vi "scale active channels.vi"(9 "input cluster":T1={"Parameters"={"FPGA Ref"=refnum, "data stream"={"data writer name"="error writer", "NS write buffer size"=16, "NS Buffer length"=0}, "FIFO Depth"=0, "Channel controls"={"FIFO channel count"=0, "active indices"=[], "active channels"=0, "channelScaling"=[], "scanivalveCount"=0, "channels"=[]}, "safetyChannels"={"oilP"=0, "airP"=0, "water"=0, "channelLimits"=[]}, "speedChannel"=0, "maxSpeedLimit"=0.0, "Torque"={"fixedOffset"=0.0, "filter"=FALSE, "fallingEdge"=FALSE, "swapEncoders"=FALSE}}, "Variables"={"Intermediary buffer"=[], "buffer position"=0, "write loop counter"=0, "NS write trigger"=0, "NS Connection status"=FALSE, "waiting for NS"=FALSE, "labAmbient"={"pressure"=0.0, "temperature"=0.0}, "scanivalvePorts"=[], "scanivalvePressures"=[], "data stream"="", "activeChannelLimitIndex"=[], "runningSpeedLimit"=0.0, "speedChannelIndex"=0, "Interlocks"={"gearboxOil"=FALSE, "bearingOil"=FALSE, "gearboxAir"=FALSE}, "interlockChannels"={"gearboxOil"=0, "bearingOil"=0, "air"=0}, "limitStates"=[]}}, 11 "raw data":sgl[](array[numeric])) -> (1 "data length":i32, 3 "Active channels":dbl[][](array[numeric]))   [LabVIEW 2018]
uses:
  Type Defs/Data processing loop data.ctl
  Type Defs/FPGA reference.ctl
  PC/type defs/channelControl.ctl
  Type Defs/channelScalingTypes.ctl
  Type Defs/scalingMethods.ctl
  ICL-LabVIEW_General/data channels/parent class/Data Channel.lvclass
  PC/type defs/channelLimitControl.ctl
  PC/type defs/limitActions.ctl
  ICL-LabVIEW_General/data channels/parent class/dataSource.ctl
  ICL-LabVIEW_General/data channels/data channels.lvlib
panel:
  out "time":dbl
  out "Data received":sgl[][](array[numeric])
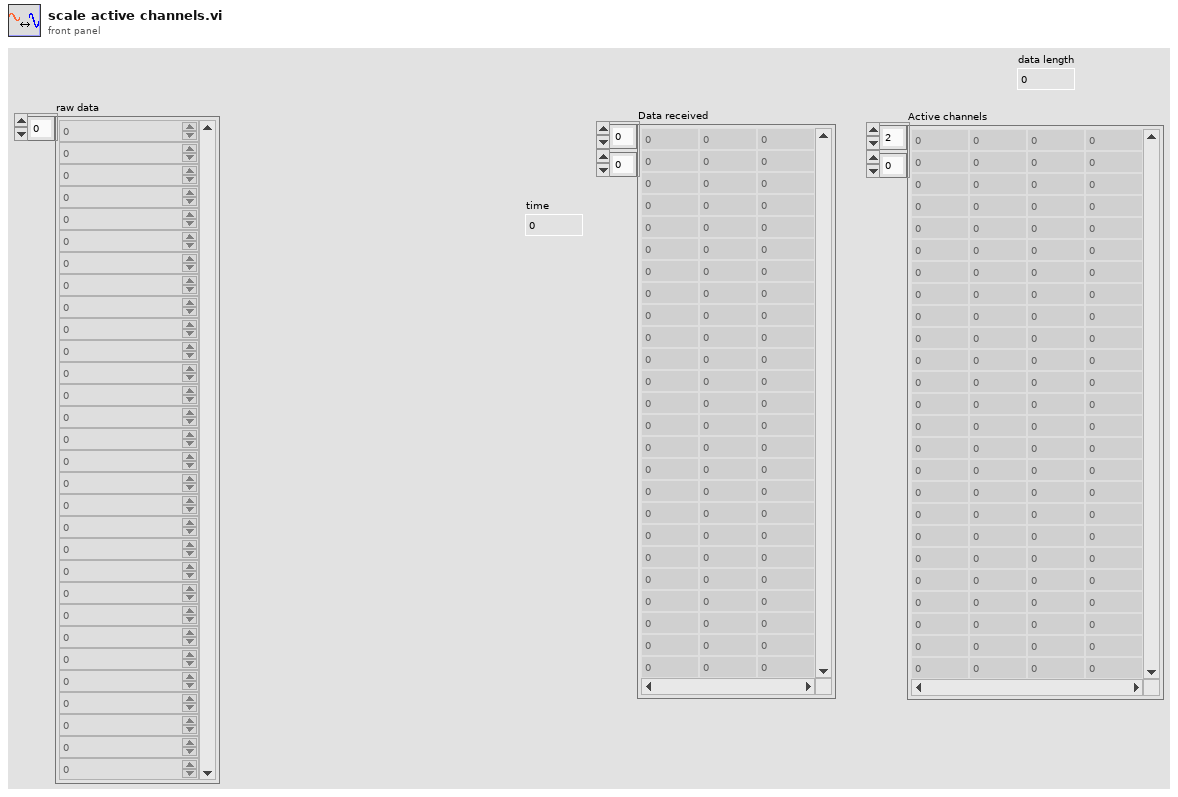
[diagram p1: front panel]
types:
  T1 = typedef "Data processing loop data.ctl" = cluster{"Parameters":cluster{"FPGA Ref":T2, "data stream":cluster{"data writer name":string, "NS write buffer size":i32, "NS Buffer length":u32}, "FIFO Depth":u32, "Channel controls":cluster{"FIFO channel count":i32, "active indices":i16[], "active channels":i32, "channelScaling":T3[], "scanivalveCount":i32, "channels":refnum<class "Data Channel.lvclass">[]}, "safetyChannels":cluster{"oilP":u16, "airP":u16, "water":u16, "channelLimits":T6[]}, "speedChannel":i32, "maxSpeedLimit":dbl, "Torque":cluster{"fixedOffset":dbl, "filter":bool, "fallingEdge":bool, "swapEncoders":bool}}, "Variables":cluster{"Intermediary buffer":dbl[][], "buffer position":u32, "write loop counter":u16, "NS write trigger":u32, "NS Connection status":bool, "waiting for NS":bool, "labAmbient":cluster{"pressure":dbl, "temperature":dbl}, "scanivalvePorts":u16[], "scanivalvePressures":dbl[], "data stream":refnum<k21>, "activeChannelLimitIndex":u16[], "runningSpeedLimit":dbl, "speedChannelIndex":i32, "Interlocks":cluster{"gearboxOil":bool, "bearingOil":bool, "gearboxAir":bool}, "interlockChannels":cluster{"gearboxOil":i32, "bearingOil":i32, "air":i32}, "limitStates":cluster{"warn":bool, "alarm":bool}[]}}
  T2 = typedef "FPGA reference.ctl" = refnum<k20>
  T3 = typedef "channelControl.ctl" = cluster{"index":u16, "active":bool, "channelType":T4, "module":u16, "terminal":u16, "channelName":string, "scalingMethod":T5, "scalingParameters":dbl[], "scaledUnits":string, "tempOffset":dbl}
  T4 = typedef "channelScalingTypes.ctl" = enum16{"calculation", "measurement", "scanivalve", "output", "digital"}
  T5 = typedef "scalingMethods.ctl" = enum16{"none", "linear", "thermocouple", "polynomial", "encoder", "RTD"}
  T6 = typedef "channelLimitControl.ctl" = cluster{"channelID":u16, "Enabled":bool, "warnValue":dbl, "limitValue":dbl, "Invert":bool, "limitAction":T7}
  T7 = typedef "limitActions.ctl" = enum16{"stop", "shutdown", "ignore"}
  T8 = typedef "data channels.lvlib/Data Channel.lvclass/dataSource.ctl" = enum16{"Not available", "FIFO", "Scanivalve", "Remote", "Calculated"}
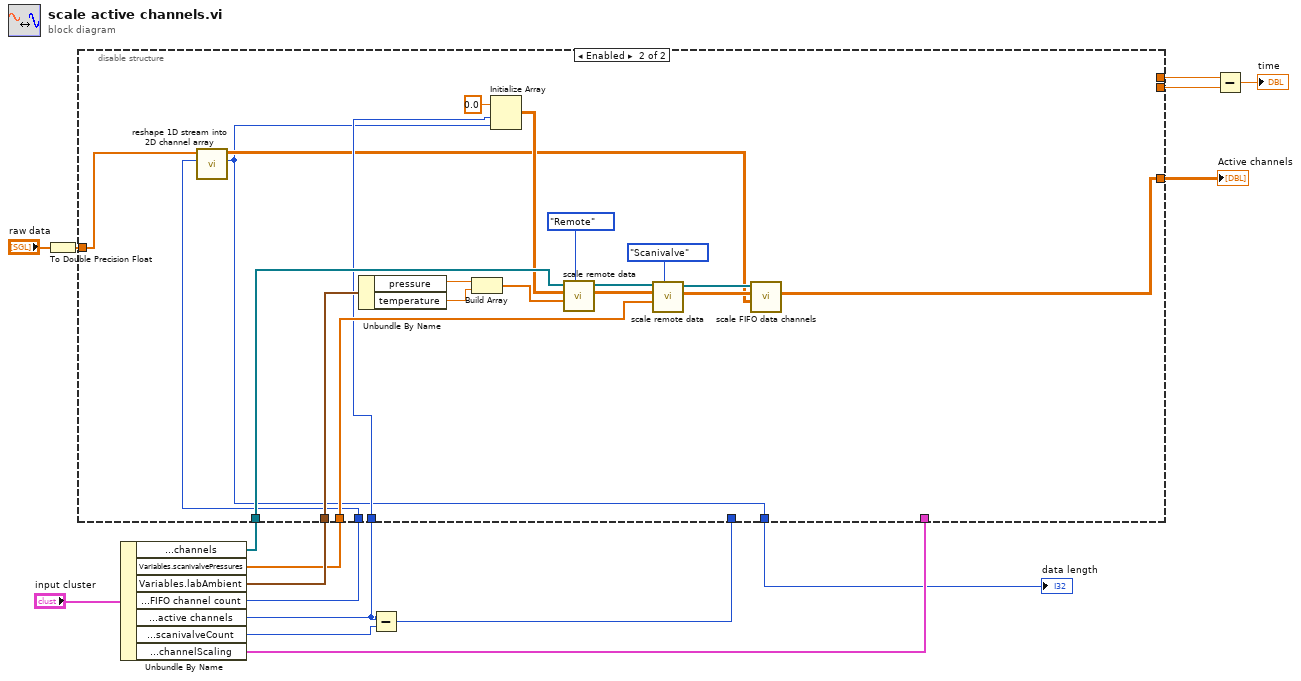
[diagram p0: block diagram]
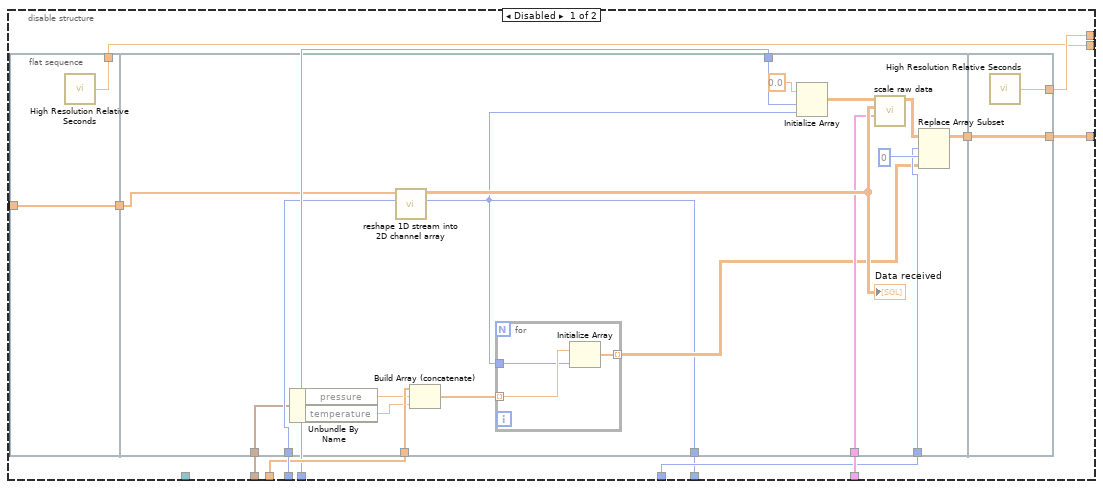
[diagram p2: hidden frame]
diagram:
  n1 = To Double Precision Float(number="raw data") -> (double precision float=w4:dbl[])
  n2 = Unbundle By Name("input cluster") -> ("Parameters.Channel controls.channels"=w3:refnum<class "Data Channel.lvclass">[], "Variables.scanivalvePressures"=w7:dbl[], "Variables.labAmbient"=w9:cluster{"pressure":dbl, "temperature":dbl}, "Parameters.Channel controls.FIFO channel count"=w10:i32, "Parameters.Channel controls.active channels"=w2:i32, "Parameters.Channel controls.scanivalveCount"=w6:i32, "Parameters.Channel controls.channelScaling"=w8:T3[])
  n3 = Subtract(x=w2, y=w6) -> (x-y=w5:i32)
  n4 = disable-structure shown="Enabled" {
    disable-tunnel: [w27 w58] -> w15
    disable-tunnel: [w26 _] -> w14
    disable-tunnel: [w25 _] -> w13
    disable-tunnel: w10 -> [w24 w67]
    disable-tunnel: w9 -> [w23 w74]
    disable-tunnel: w8 -> [w22 _]
    disable-tunnel: w7 -> [w21 w70]
    disable-tunnel: w2 -> [w20 w65]
    disable-tunnel: w5 -> [w19 _]
    disable-tunnel: w4 -> [w18 w68]
    disable-tunnel: w3 -> [_ w69]
    disable-tunnel: [w17 w57] -> w1
    frame Disabled {
      n5 = flat-sequence {
        tunnel: w18 -> [w31]
        tunnel: [w31] -> w29
        tunnel: [w30] -> w25
        tunnel: w29 -> [w49]
        tunnel: [w44] -> w28
        tunnel: w24 -> [w43]
        tunnel: w23 -> [w42]
        tunnel: w22 -> [w41]
        tunnel: w21 -> [w40]
        tunnel: w20 -> [w36]
        tunnel: w19 -> [w34]
        tunnel: [w32] -> w17
        tunnel: [w54] -> w27
        tunnel: w28 -> [w54]
        tunnel: [w53] -> w26
        frame #0 {
          n6 = call <vilib>:"High Resolution Relative Seconds.vi"() -> ("relative seconds"=w30:dbl)
        }
        frame #1 {
          n7 = Unbundle By Name(w42) -> ("pressure"=w39:dbl, "temperature"=w38:dbl)
          n8 = call "reshape 1D stream into 2D channel array.vi"("FIFIO channel count"=w43, "1D datastream in"=w49) -> ("dataPoints"=w32:i32, "2D data array out"=w48:dbl[][])  [unwired: 8 in]
          "Data received" <- w48
          n9 = Build Array (concatenate)(w40, w39, w38) -> (w37:dbl[])
          n10 = for {
            tunnel: w37 -> [w52] mode=indexing
            tunnel: w32 -> [w51]
            tunnel: [w50] -> w33 mode=indexing
            n11 = Initialize Array(w52, w51) -> (w50:dbl[])
          }
          n12 = Initialize Array(0.0 ("raw data"), w36, w32) -> (w46:dbl[][])
          n13 = call "scale raw data.vi"("channelScaling"=w41, "raw data"=w48, "scaled data"=w46) -> ("scaled data"=w45:dbl[][])  [unwired: 8 in]
          n14 = Replace Array Subset(array=w45, new element=w33, index (row)=w34, index (col)=0 ("disabled index (row)")) -> (w44:dbl[][])
        }
        frame #2 {
          n15 = call <vilib>:"High Resolution Relative Seconds.vi"() -> ("relative seconds"=w53:dbl)
        }
      }
    }
    frame Enabled {
      n16 = call "reshape 1D stream into 2D channel array.vi"("FIFIO channel count"=w67, "1D datastream in"=w68) -> ("dataPoints"=w57:i32, "2D data array out"=w59:dbl[][])  [unwired: 8 in]
      n17 = Unbundle By Name(w74) -> ("pressure"=w73:dbl, "temperature"=w72:dbl)
      n18 = Build Array(w73, w72) -> (w71:dbl[])
      n19 = Initialize Array(0.0 ("element"), w65, w57) -> (w64:dbl[][])
      n20 = call "scale remote data.vi"("dataSource"=dataSource."Remote", "remoteData"=w71, "unscaledRemoteData"=w64, "channels"=w69) -> ("scaledRemoteData"=w62:dbl[][], "channels out"=w63:refnum<class "Data Channel.lvclass">[])  [unwired: 6 in]
      n21 = call "scale remote data.vi"("dataSource"=dataSource."Scanivalve", "remoteData"=w70, "unscaledRemoteData"=w62, "channels"=w63) -> ("scaledRemoteData"=w60:dbl[][], "channels out"=w61:refnum<class "Data Channel.lvclass">[])  [unwired: 6 in]
      n22 = call "scale FIFO data channels.vi"("FIFO data"=w59, "empty scaled data"=w60, "dataChannels"=w61) -> ("scaled data"=w58:dbl[][])  [unwired: 8 in]
    }
  }
  "Active channels" <- w15
  "data length" <- w1
  n23 = Subtract(x=w14, y=w13) -> (x-y=→"time":dbl)
